vi "Create Boolean Tags.vi"(8 "error in (no error)":errorcluster, 10 "All Boolean Tags":string[](array[string]), 11 "Tag Category":string) -> (0 "Error Array":errorcluster[](array[cluster]))   [LabVIEW 2018, in "Feed Module.lvlib" / "Feed Module Engine.lvlib"]
uses:
  Feed Module Engine.lvlib
  Tag VIs/Tag FGV Operation Enum.ctl
  support/Support Library.lvlib
  Shared Variables/Dynamic Shared Variables.lvlib
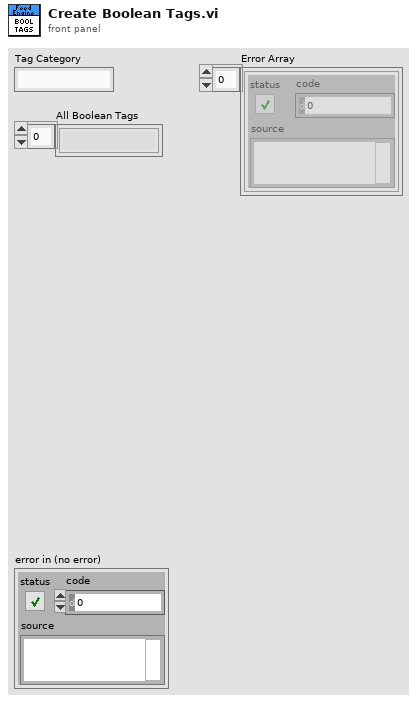
[diagram p1: front panel]
types:
  T1 = cluster{"enable? (F)":bool, "name":string, "alarm on":bool, "priority":u32, "ack type":enum16{"Auto", "User", "None", "Each Occurrence"}, "area":string, "description":string, "log? (T)":bool}
  T2 = enum32{"u32BitField", "bool", "double", "string", "int8", "uint8", "int16", "uint16", "int32", "uint32", "int64", "uint64", "single", "double waveform", "int16 waveform", "array of boolean", "array of int8", "array of uint8", "array of int16", "array of uint16", "array of int32", "array of uint32", "array of int64", "array of uint64", "array of single", "array of double", "array of double waveform", "array of int16 waveform", "array of string", "variant", "timestamp", "fixed point", "custom"}
  T3 = typedef "Tag FGV Operation Enum.ctl" = enum16{"Init", "Set Notification Queue", "Create Tag", "Commit", "Write Tag (Numeric)", "Write Tag (Boolean)", "Read All Tags", "Read One Tag", "Delete Tag Category", "Set Alarm Parameters (Numeric)", "Set Alarm Parameters (Boolean)", "Enable All Alarms", "Disable All Alarms", "Delete All Tags", "Read Alarms", "Ack Alarm", "Read Alarm Parameters (Numeric)", "Read Alarm Parameters (Boolean)"}
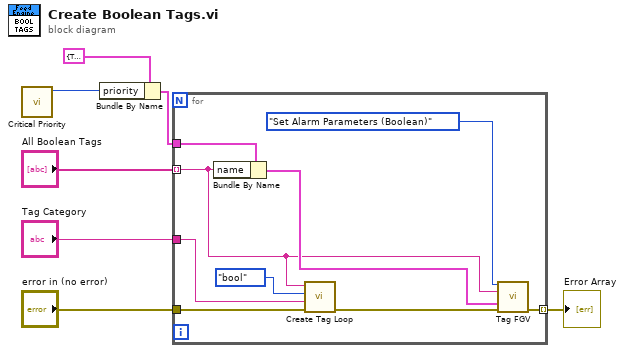
[diagram p0: block diagram]
diagram:
  n1 = call "Critical Priority.vi"() -> ("critical priority"=w2:i32)  [unwired: 11 in]
  n2 = Bundle By Name(cluster=T1 {"enable? (F)"=TRUE, "name"="Boolean", "alarm on"=TRUE, "priority"=1, "ack type"=enum."Each Occurrence", "area"="a", "description"="", "log? (T)"=TRUE} ("Boolean alarm settings"), "priority"=w2) -> (w1:T1)
  n3 = for {
    tunnel: w1 -> [w16]
    tunnel: [w15] -> w5 mode=indexing
    tunnel: "All Boolean Tags" -> [w11] mode=indexing
    tunnel: "error in (no error)" -> [w9]
    tunnel: "Tag Category" -> [w10]
    n4 = Bundle By Name(cluster=w16, "name"=w11) -> (w14:T1)
    n5 = call "Create Tag Loop.vi"("error in (no error)"=w9, "Tag Category"=w10, "data type"=T2."bool", "Tag Name"=w11) -> ("error out"=w8:errorcluster)  [unwired: 7 in]
    n6 = call "Tag FGV.vi"("Operation"=Tag_FGV_Operation_Enum."Set Alarm Parameters (Boolean)", "Tag Name"=w11, "Data"=w14, "error in (no error)"=w8) -> ("error out"=w15:errorcluster)  [unwired: 4 in, 7 out]
  }
  "Error Array" <- w5
